vi "Global Constants.vi"() -> ()   [LabVIEW 2017]
panel:
  in  "Elevator fudge factor":dbl=1000.0
  in  "Elevator acceptable range":dbl=1000.0
  in  "Elevator Loop Iteration Time":dbl=5.0
  in  "Yaw acceptable turn range":dbl=5.0
  in  "Drive Loop Iteration Time":dbl=5.0
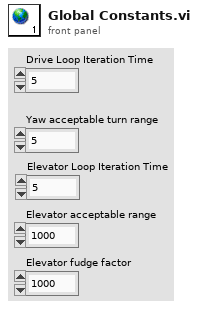
[diagram p1: front panel]
diagram:
